vi "Connect.vi"(8 "Error In":errorcluster, 11 "object in":refnum<class "PXI-5441.lvclass">) -> (0 "Error Out":errorcluster, 3 "object out":refnum<class "PXI-5441.lvclass">)   [LabVIEW 2023, in "HAL.lvlib" / "PXI-5441.lvlib" / "PXI-5441.lvclass"]
uses:
  PXI-5441.lvclass
  PXI-5441.lvclass/PXI-5441.ctl
  FGEN_class/states/IStates_interface/IStates.lvclass
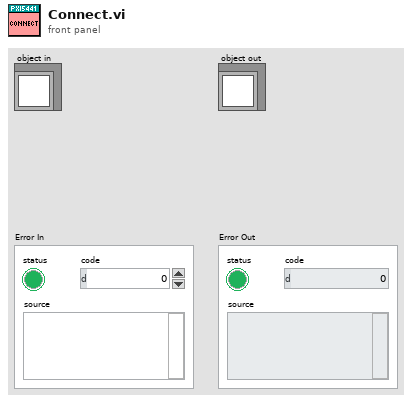
[diagram p1: front panel]
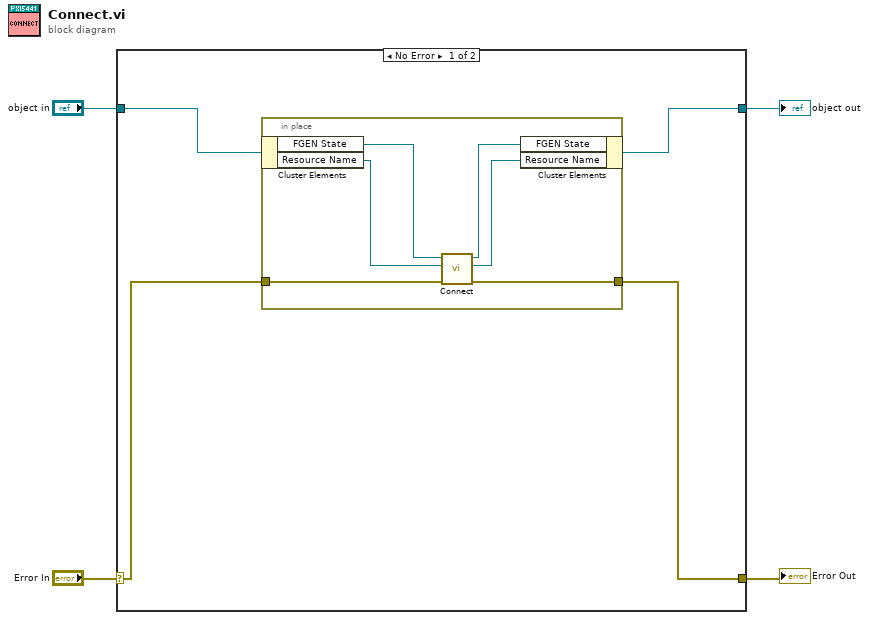
[diagram p0: block diagram]
diagram:
  n1 = case shown="No Error" "Error In" {
    selector: "Error In" -> [w8 w16]
    tunnel: [w5 w16] -> w3
    tunnel: [w6 w15] -> w1
    tunnel: "object in" -> [w7 w15]
    frame No Error {
      n2 = in-place {
        in-place-border: w8 -> [w14]
        in-place-border: [w11] -> w5
        n3 = in-place-cluster #1(w7) -> ("FGEN State"=w13:refnum<class "IStates.lvclass">, "Resource Name"=w10:refnum<k15>)
        n4 = call-dynamic "Connect.vi"("Error In"=w14, "Resource Name"=w10, "object in"=w13) -> ("Error Out"=w11:errorcluster, "Resource Name out"=w9:refnum<k15>, "object out"=w12:refnum<class "IStates.lvclass">)  [unwired: 6 in]
        n5 = in-place-cluster #1("FGEN State"=w12, "Resource Name"=w9) -> (w6:refnum<class "PXI-5441.lvclass">)
      }
    }
    frame Error {
    }
  }
  "Error Out" <- w3
  "object out" <- w1
